vi "Acquire Data from Hardware.vi"(8 "error in (no error)":cluster{"状态":bool, "代码":i32, "源":string} caption="错误输入（无错误）", 11 "硬件配置":T1) -> (0 "error out":cluster{"状态":bool, "代码":i32, "源":string} caption="错误输出", 2 "图形数据":waveform(dbl)[](array[waveform]))   [LabVIEW 2013]
doc: "按硬件配置输入中的信号类型，生成采样波形。"
uses:
  controls/HW Configuration.ctl
  controls/Simulated Signal Type.ctl
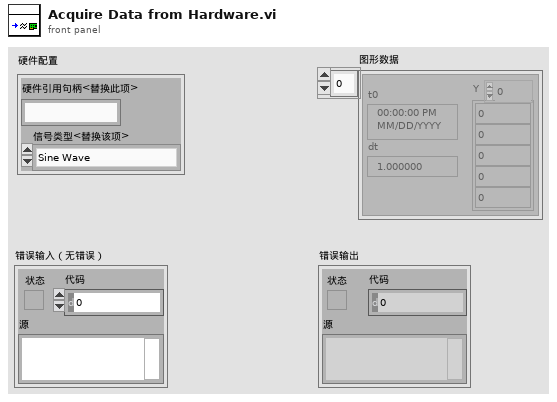
[diagram p1: front panel]
types:
  T1 = typedef "HW Configuration.ctl" = cluster{"硬件引用句柄<替换此项>":string, "信号类型<替换该项>":T2}
  T2 = typedef "Simulated Signal Type.ctl" = enum16{"Sine Wave", "Square Wave"}
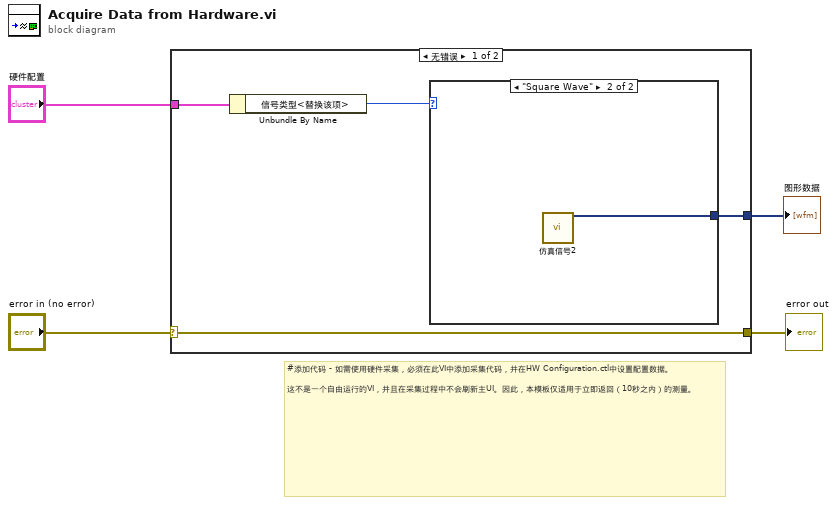
[diagram p0: block diagram]
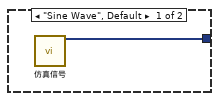
[diagram p2: hidden frame]
diagram:
  # "#添加代码 - 如需使用硬件采集，必须在此VI中添加采集代码，并在HW Configuration.ctl中设置配置数据。\n\n这不是一个自由运行的VI，并且在采集过程中不会刷新主UI。因此，本模板仅适用于立即返回（10秒之内）的测量。"
  n1 = case shown="无错误" "error in (no error)" {
    selector: "error in (no error)" -> [w8 w11]
    tunnel: [w8 w11] -> w3
    tunnel: "硬件配置" -> [w7 _]
    tunnel: [w6 _] -> w1
    frame No Error {
      n2 = Unbundle By Name(w7) -> ("信号类型<替换该项>"=w5:T2)
      n3 = case shown="\"Square Wave\"" w5 {
        tunnel: [w9 w10] -> w6
        frame "Sine Wave", Default {
          n4 = call "仿真信号"() -> ("Sine"=w9:dynamicdata)  [unwired: 14 in, 1 out]
        }
        frame "Square Wave" {
          n5 = call "仿真信号2"() -> ("Square"=w10:dynamicdata)  [unwired: 14 in, 1 out]
        }
      }
    }
    frame Error {
    }
  }
  "error out" <- w3
  "图形数据" <- w1
